vi "read.vi"(8 "error in (no error)":errorcluster, 11 "SimAnalogHardware in":refnum<class "SimAnalogHardware.lvclass">) -> (0 "error out":errorcluster, 2 "outputs":u16[][](array[numeric]), 3 "SimAnalogHardware out":refnum<class "SimAnalogHardware.lvclass">)   [LabVIEW 2017, in "SimAnalogHardware.lvclass"]
doc: "Read data from the instrument"
uses:
  SimAnalogHardware.lvclass
  support/my_global.vi
panel:
  # "2d array of u16"
  # "If the number is greater than 32767 that means\nthe actual value is negativ and it is complementary code.\nBy subtracting 65536 this number will be converted to signed\ninteger."
  # "https://knowledge.ni.com/KnowledgeArticleDetails?id=kA00Z0000019YLoSAM&l=de-DE"
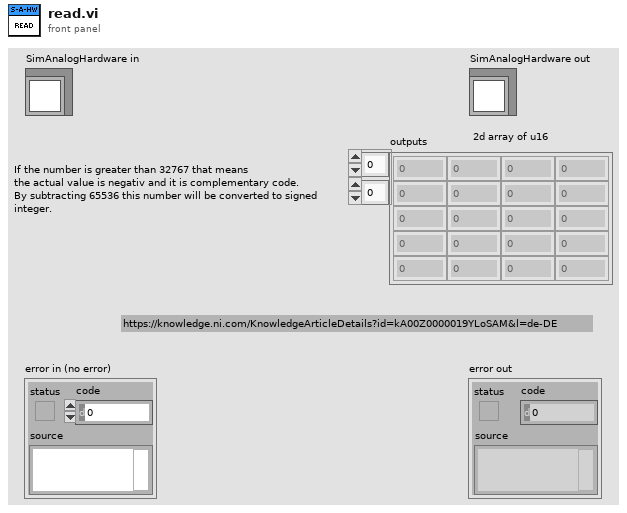
[diagram p1: front panel]
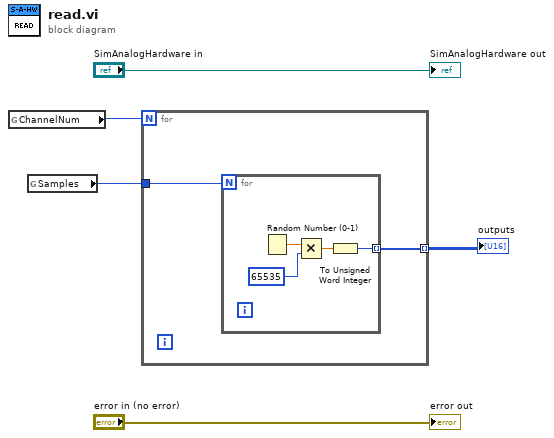
[diagram p0: block diagram]
diagram:
  n1 = global read "my_global.vi" "ChannelNum"() -> (w3:u32)
  n2 = global read "my_global.vi" "Samples"() -> (w2:u32)
  n3 = for {
    N: w3 -> [_]
    tunnel: w2 -> [w7]
    tunnel: [w6] -> w1 mode=indexing
    n4 = for {
      N: w7 -> [_]
      tunnel: [w8] -> w6 mode=indexing
      n5 = Random Number (0-1)() -> (number: 0 to 1=w11:dbl)
      n6 = Multiply(x=w11, y=u16 65535) -> (x*y=w9:dbl)
      n7 = To Unsigned Word Integer(number=w9) -> (unsigned 16bit integer=w8:u16)
    }
  }
  "outputs" <- w1
  "error out" <- "error in (no error)"
  "SimAnalogHardware out" <- "SimAnalogHardware in"
